vi "PolySetIcon.vi"   [LabVIEW 2020]
types:
  T1 = cluster{"VIPath":path, "Menu Name":string, "Selector Name":string}[]
  T2 = typedef "imagedata.ctl" = cluster{"image type":i32, "image depth":i32, "image":u8[], "mask":u8[], "colors":u32[], "Rectangle":cluster{"left":i16, "top":i16, "right":i16, "bottom":i16}}
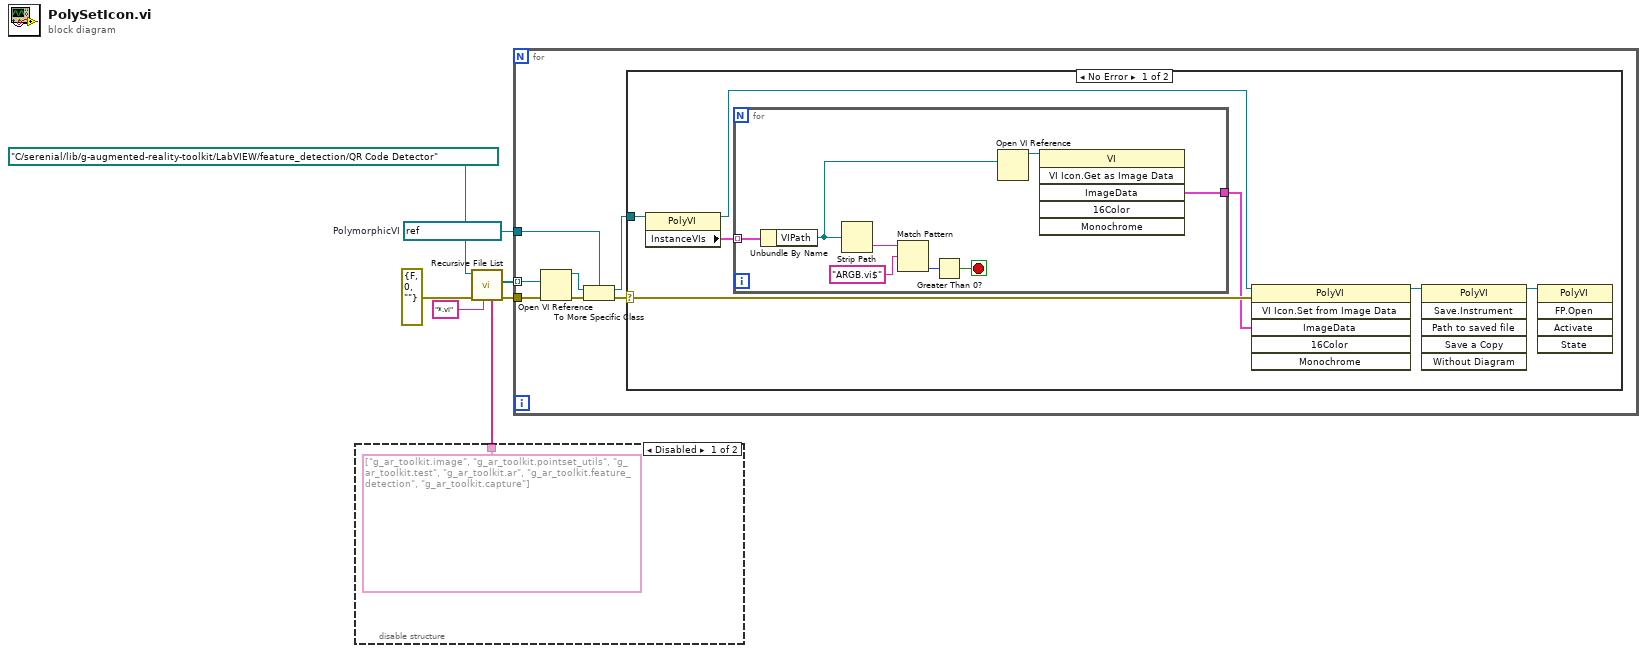
[diagram p0: block diagram]
diagram:
  w4 = refnum<vi> refnum  # PolymorphicVI
  n1 = disable-structure shown="Disabled" {
    disable-tunnel: [string[] ["g_ar_toolkit.image", "g_ar_toolkit.pointset_utils", "g_ar_toolkit.test", "g_ar_toolkit.ar", "g_ar_toolkit.feature_detection", "g_ar_toolkit.capture"] ("Folders to Exclude") _] -> w1
    frame Disabled {
    }
    frame Enabled {
    }
  }
  n2 = call <vilib>:"Recursive File List.vi"("Folders to Exclude"=w1, "pattern"="*.vi", "error in (no error)"=errorcluster {"status"=FALSE, "code"=0, "source"=""} ("error out"), "Folder Path"=path "C:/serenial/lib/g-augmented-reality-toolkit/LabVIEW/feature_detection/QR Code Detector") -> ("error out"=w7:errorcluster, "All Files in Dir"=w6:path[])  [unwired: 3 in, 3 out]
  n3 = for {
    tunnel: w7 -> [w15]
    tunnel: w6 -> [w14] mode=indexing
    tunnel: w4 -> [w13]
    n4 = Open VI Reference(vi path=w14, error in (no error)=w15) -> (vi reference=w12:refnum<vi>, error out=w11:errorcluster)  [unwired: 4 in]
    n5 = To More Specific Class(target class=w13, reference=w12, error in=w11) -> (specific class reference=w9:refnum<vi>, error out=w10:errorcluster)
    n6 = case shown="No Error" w10 {
      selector: w10 -> [w22 _]
      tunnel: w9 -> [w21 _]
      frame No Error {
        n7 = property class="PolyVI"(reference=w21) -> (reference out=w20:refnum<vi>, "InstanceVIs"=w19:T1)  [unwired: 1 in, 1 out]
        n8 = for {
          tunnel: w19 -> [w30] mode=indexing
          tunnel: [w25] -> w18
          stop <- w24 stop-if-true
          n9 = Unbundle By Name(w30) -> ("VIPath"=w26:path)
          n10 = Strip Path(path=w26) -> (name=w29:string)  [unwired: 1 out]
          n11 = Match Pattern(string=w29, regular expression="ARGB.vi$") -> (offset past match=w27:i32)  [unwired: 1 in, 3 out]
          n12 = Greater Than 0?(x=w27) -> (x > 0?=w24:bool)
          n13 = Open VI Reference(vi path=w26) -> (vi reference=w23:refnum<vi>)  [unwired: 5 in, 1 out]
          n14 = invoke class="VI" method="VI Icon.Get as Image Data"(reference=w23) -> ("ImageData"=w25:T2)  [unwired: 5 in, 5 out]
        }
        n15 = invoke class="PolyVI" method="VI Icon.Set from Image Data"(reference=w20, error in=w22, "ImageData"=w18) -> (reference out=w17:refnum<vi>)  [unwired: 3 in, 5 out]
        n16 = invoke class="PolyVI" method="Save.Instrument"(reference=w17) -> (reference out=w16:refnum<vi>)  [unwired: 5 in, 5 out]
        n17 = invoke class="PolyVI" method="FP.Open"(reference=w16) -> ()  [unwired: 4 in, 5 out]
      }
      frame Error {
      }
    }
  }
